vi "S2C_VAR_DragEnd.vi"(8 "Error In":errorcluster, 11 "CtrlRef":refnum<vi>) -> (0 "Error Out":errorcluster)   [LabVIEW 2015]
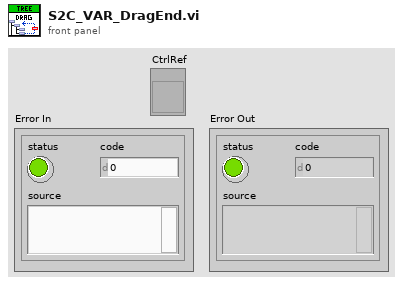
[diagram p1: front panel]
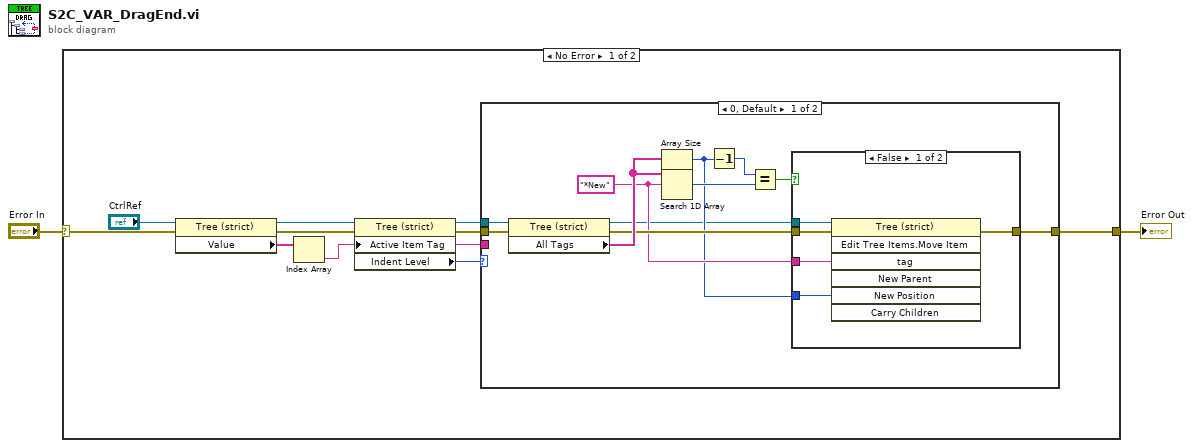
[diagram p0: block diagram]
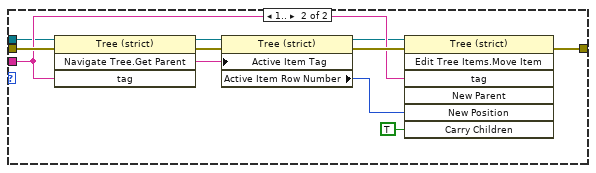
[diagram p3: hidden frame]
diagram:
  n1 = case shown="No Error" "Error In" {
    selector: "Error In" -> [w7 w41]
    tunnel: [w3 w41] -> w1
    frame No Error {
      n2 = property on="Property Node" class="Tree (strict)"(reference="CtrlRef", error in=w7) -> (reference out=w5:refnum<vi>, error out=w11:errorcluster, "Value"=w12:string[])
      n3 = Index Array(array=w12) -> (element=w8:string)  [unwired: 1 in]
      n4 = property on="Property Node" class="Tree (strict)"(reference=w5, error in=w11, "Active Item Tag"=w8) -> (reference out=w4:refnum<vi>, error out=w10:errorcluster, "Indent Level"=w9:i32)
      n5 = case shown="0, Default" w9 {
        tunnel: [w23 w34] -> w3
        tunnel: w10 -> [w15 w40]
        tunnel: w8 -> [_ w36]
        tunnel: w4 -> [w14 w32]
        frame 0, Default {
          w18 = "*New" ("element")
          n6 = property on="Property Node" class="Tree (strict)"(reference=w14, error in=w15) -> (reference out=w13:refnum<vi>, error out=w20:errorcluster, "All Tags"=w22:string[])
          n7 = Array Size(array=w22) -> (size(s)=w16:i32)
          n8 = Search 1D Array(1D array=w22, element=w18) -> (index of element=w21:i32)  [unwired: 1 in]
          n9 = Decrement(x=w16) -> (x-1=w17:i32)
          n10 = Equal?(x=w17, y=w21) -> (x = y?=w19:bool)
          n11 = case shown="False" w19 {
            tunnel: w20 -> [w28 w29]
            tunnel: [w27 w29] -> w23
            tunnel: w18 -> [w26 _]
            tunnel: w16 -> [w25 _]
            tunnel: w13 -> [w24 _]
            frame False {
              n12 = invoke on="Invoke Node" class="Tree (strict)" method="Edit Tree Items.Move Item"(reference=w24, error in=w28, "tag"=w26, "New Position"=w25) -> (error out=w27:errorcluster)  [unwired: 3 in, 6 out]
            }
            frame True {
            }
          }
        }
        frame 1.. {
          n13 = invoke on="Invoke Node" class="Tree (strict)" method="Navigate Tree.Get Parent"(reference=w32, error in=w40, "tag"=w36) -> (reference out=w31:refnum<vi>, error out=w39:errorcluster, "Navigate Tree:Get Parent"=w38:string)  [unwired: 1 in, 1 out]
          n14 = property on="Property Node" class="Tree (strict)"(reference=w31, error in=w39, "Active Item Tag"=w38) -> (reference out=w30:refnum<vi>, error out=w37:errorcluster, "Active Item Row Number"=w35:i32)
          n15 = invoke on="Invoke Node" class="Tree (strict)" method="Edit Tree Items.Move Item"(reference=w30, error in=w37, "tag"=w36, "New Position"=w35, "Carry Children"=TRUE ("Carry Children?")) -> (error out=w34:errorcluster)  [unwired: 2 in, 6 out]
        }
      }
    }
    frame Error {
    }
  }
  "Error Out" <- w1
